vi "FT02Parameters.vi"() -> ()   [LabVIEW 2012]
panel:
  in  "FT02Parameters":T1={"baudrate"=9600, "Port Com"=0, "Tag"=0, "FlowLimit"=0.0, "IDH"=0, "IDM"=0, "IDL"=0, "IDS"=0}
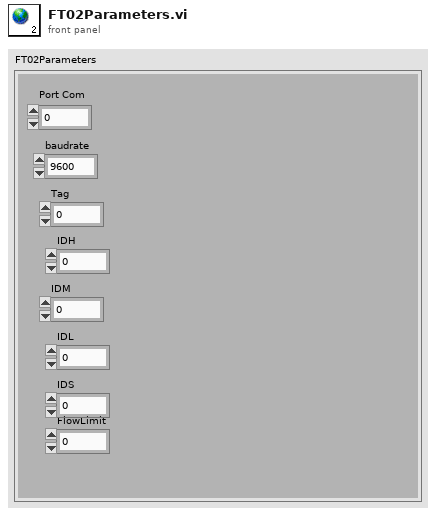
[diagram p1: front panel]
types:
  T1 = cluster{"baudrate":i32, "Port Com":i32, "Tag":u32, "FlowLimit":dbl, "IDH":u8, "IDM":u8, "IDL":u8, "IDS":u8}
diagram:
